vi "CleanAndGetNames.vi"(6 "Status":refnum<vi>, 8 "error in":errorcluster, 11 "Working Dir":path) -> (0 "error out":errorcluster, 1 "Deleted files":string[](array[string]), 2 "filenames":string[](array[string]), 3 "Working Dir Out":path)   [LabVIEW 2022 SP3]
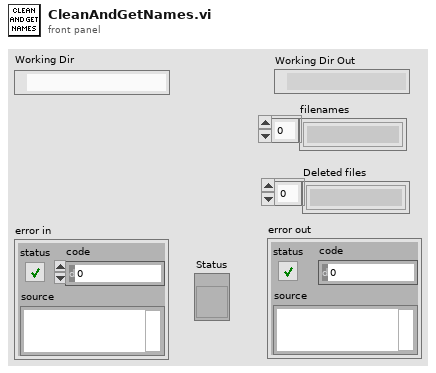
[diagram p1: front panel]
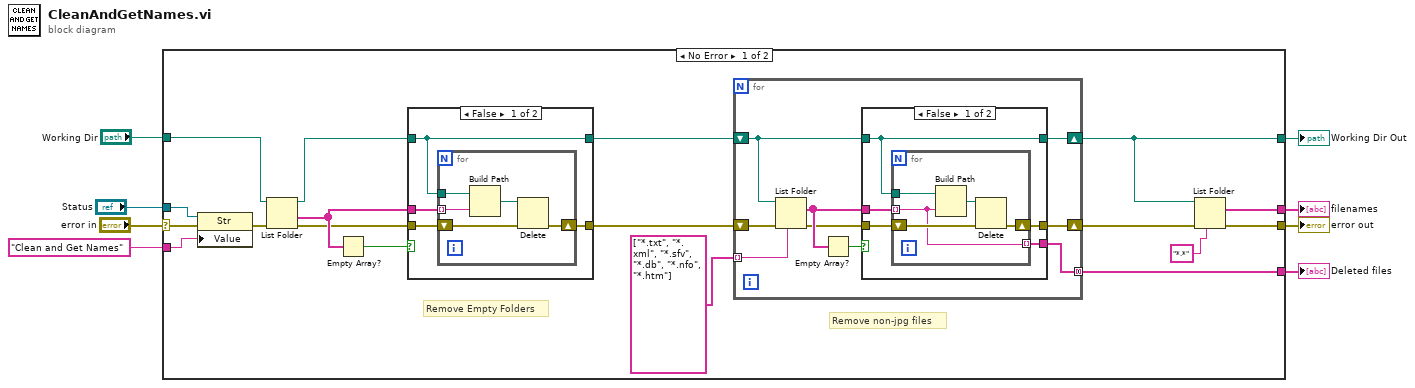
[diagram p0: block diagram]
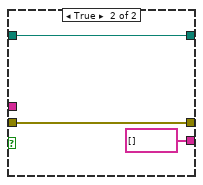
[diagram p2: hidden frame]
diagram:
  n1 = case shown="No Error" "error in" {
    selector: "error in" -> [w10 w60]
    tunnel: "Working Dir" -> [w21 w61]
    tunnel: [w17 w61] -> w7
    tunnel: [w16 w60] -> w6
    tunnel: [w15 _] -> w5
    tunnel: [w14 _] -> w4
    tunnel: "Status" -> [w12 _]
    tunnel: "Clean and Get Names" ("Value") -> [w11 _]
    frame No Error {
      # "Remove non-jpg files"
      # "Remove Empty Folders"
      n2 = property class="Str"(reference=w12, error in=w10, "Value"=w11) -> (error out=w13:errorcluster)  [unwired: 1 out]
      n3 = List Folder(path=w21, error in=w13) -> (path out=w20:path, folder names=w25:string[], error out=w24:errorcluster)  [unwired: 2 in, 1 out]
      n4 = Empty Array?(array=w25) -> (empty?=w26:bool)
      n5 = case shown="False" w26 {
        tunnel: w25 -> [w52 _]
        tunnel: w20 -> [w49 w58]
        tunnel: w24 -> [w51 w59]
        tunnel: [w50 w59] -> w22
        tunnel: [w49 w58] -> w23
        frame False {
          n6 = for {
            tunnel: w52 -> [w55] mode=indexing
            tunnel: w49 -> [w56]
            shift-right: [w53] -> w50
            shift-left: w51 -> [w54]
            n7 = Build Path(base path=w56, name or relative path=w55) -> (appended path=w57:path)
            n8 = Delete(path (use dialog)=w57, error in=w54) -> (error out=w53:errorcluster)  [unwired: 3 in, 2 out]
          }
        }
        frame True {
        }
      }
      n9 = for {
        shift-right: [w29] -> w18
        shift-left: w22 -> [w35]
        tunnel: string[] ["*.txt", "*.xml", "*.sfv", "*.db", "*.nfo", "*.htm"] -> [w34] mode=indexing
        shift-right: [w28] -> w17
        shift-left: w23 -> [w33]
        tunnel: [w27] -> w15 mode=concatenating
        n10 = List Folder(path=w33, pattern=w34, error in=w35) -> (filenames=w31:string[], error out=w30:errorcluster)  [unwired: 1 in, 2 out]
        n11 = Empty Array?(array=w31) -> (empty?=w32:bool)
        n12 = case shown="False" w32 {
          tunnel: w31 -> [w40 _]
          tunnel: w33 -> [w37 w47]
          tunnel: w30 -> [w39 w48]
          tunnel: [w38 w48] -> w29
          tunnel: [w37 w47] -> w28
          tunnel: [w36 string[] []] -> w27
          frame False {
            n13 = for {
              tunnel: w40 -> [w41] mode=indexing
              tunnel: w37 -> [w44]
              shift-right: [w42] -> w38
              shift-left: w39 -> [w43]
              tunnel: [w41] -> w36 mode=indexing
              n14 = Build Path(base path=w44, name or relative path=w41) -> (appended path=w45:path)
              n15 = Delete(path (use dialog)=w45, error in=w43) -> (error out=w42:errorcluster)  [unwired: 3 in, 2 out]
            }
          }
          frame True {
          }
        }
      }
      n16 = List Folder(path=w17, pattern="*.*", error in=w18) -> (filenames=w14:string[], error out=w16:errorcluster)  [unwired: 1 in, 2 out]
    }
    frame Error {
    }
  }
  "Working Dir Out" <- w7
  "error out" <- w6
  "Deleted files" <- w5
  "filenames" <- w4
